vi "Explain exception code.vi"(10 "exception":i32, 11 "Job type":refnum<class "Job.lvclass">) -> (1 "exception message":string, 2 "exception dup":i32, 3 "warning?":bool)   [LabVIEW 2013, in "openCronJob.lvlib" / "Job.lvclass"]
uses:
  Job.lvclass
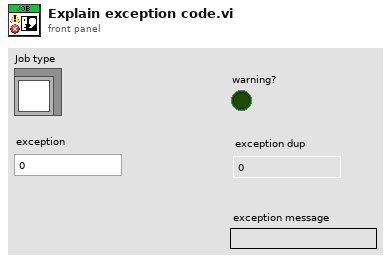
[diagram p1: front panel]
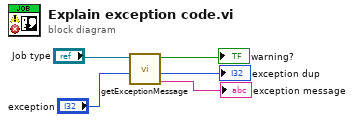
[diagram p0: block diagram]
diagram:
  n1 = call-dynamic "getExceptionMessage.vi"("exception"="exception", "Job in"="Job type") -> ("exception message"=→"exception message":string, "exception dup"=→"exception dup":i32, "warning?"=→"warning?":bool)  [unwired: 7 in]
